vi "Quick Load Audio File.vi"   [LabVIEW 2020, in "G-Audio.lvlib"]
doc: "<b>This VI is polymorphic.</b>\n\nA single VI method to load an entire audio file from disk. The audio data will be returned as an I16 waveform array.\n\nNote this method is faster than reading audio chunks in a loop, but can result in higher peak memory allocation. If the file is very large, LabVIEW may run out of memory.\n\n<b>Path</b> can be a standard path type, or a UTF-8 encoded string.\n\nSupported codecs: flac, mp3, ogg (vorbis), and wav."
uses:
  G-Audio.lvlib
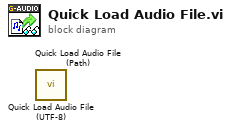
[diagram p0: block diagram]
diagram:
  n1 = call "Quick Load Audio File (UTF-8).vi"() -> ()  [unwired: 6 in, 6 out]
  n2 = call "Quick Load Audio File (Path).vi"() -> ()  [unwired: 6 in, 6 out]
